vi "Lookup Form Field.vi"(8 "error in (no error)":errorcluster, 10 "Name":string, 11 "Request in":refnum<class "Request.lvclass">) -> (0 "error out":errorcluster, 1 "Exists":bool, 2 "Field":refnum<class "FormField.lvclass">, 3 "Request out":refnum<class "Request.lvclass">)   [LabVIEW 2020, in "HTTP Utils.lvlib" / "Request.lvclass"]
uses:
  Request.lvclass
  FormField/FormField.lvclass
  Request.lvclass/Request.ctl
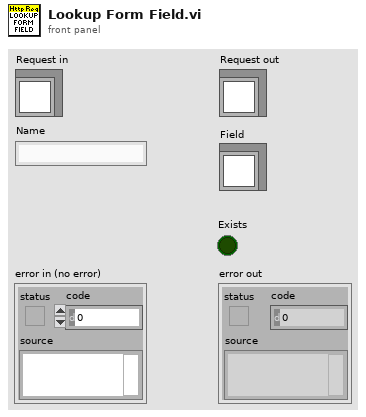
[diagram p1: front panel]
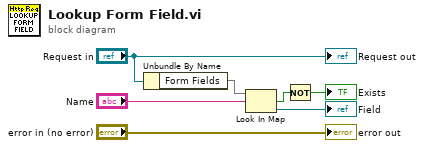
[diagram p0: block diagram]
diagram:
  n1 = Unbundle By Name("Request in") -> ("Form Fields"=w7:map{string, refnum<class "FormField.lvclass">})
  n2 = Look In Map(map=w7, key="Name") -> (key not found?=w5:bool, value=→"Field":refnum<class "FormField.lvclass">)  [unwired: 1 in]
  n3 = Not(x=w5) -> (.not. x?=→"Exists":bool)
  "error out" <- "error in (no error)"
  "Request out" <- "Request in"
